vi "Create User Events.vi"(8 "error in":errorcluster) -> (0 "error out":errorcluster, 3 "User Events Ref":T1)   [LabVIEW 2014, in "Events Lib.lvlib"]
uses:
  Events Lib.lvlib
  Events TypeDef.ctl
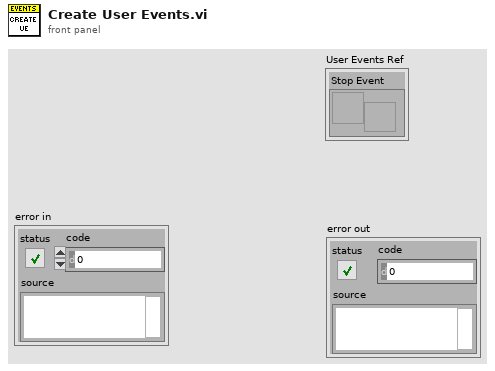
[diagram p1: front panel]
types:
  T1 = typedef "Events Lib.lvlib/Events TypeDef.ctl" = cluster{"Stop Event":refnum<user-event>}
  T2 = enum16{"Create Events", "Get Events", "Destroy Events"}
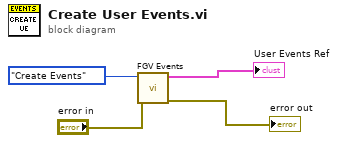
[diagram p0: block diagram]
diagram:
  n1 = call "FGV Events.vi"("error in"="error in", "Action"=T2."Create Events") -> ("error out"=→"error out":errorcluster, "Cluster"=→"User Events Ref":T1)  [unwired: 8 in]
